vi "MoveZ.vi"(0 "Speed (unit/s)":dbl min=0.0 max=1500.0, 1 "Relative/Absolute\nPosition":enum16{"Relative", "Absolute"}(ring), 2 "connection refnum in":refnum<k5>, 5 "Speed Units":enum16{"mm", "µm"}(ring), 7 "Target Position":dbl, 9 "Target Units":enum16{"mm", "µm"}(ring), 11 "error in":errorcluster) -> (4 "connection refnum out z":refnum<k5>, 6 "approx move time (ms)":i32, 15 "error out":errorcluster)   [LabVIEW 2023]
doc: "Move in a fixed step to a target location in the Z direction"
uses:
  GlobalVarsNetwork.vi
panel:
  in  "Stop Button":bool
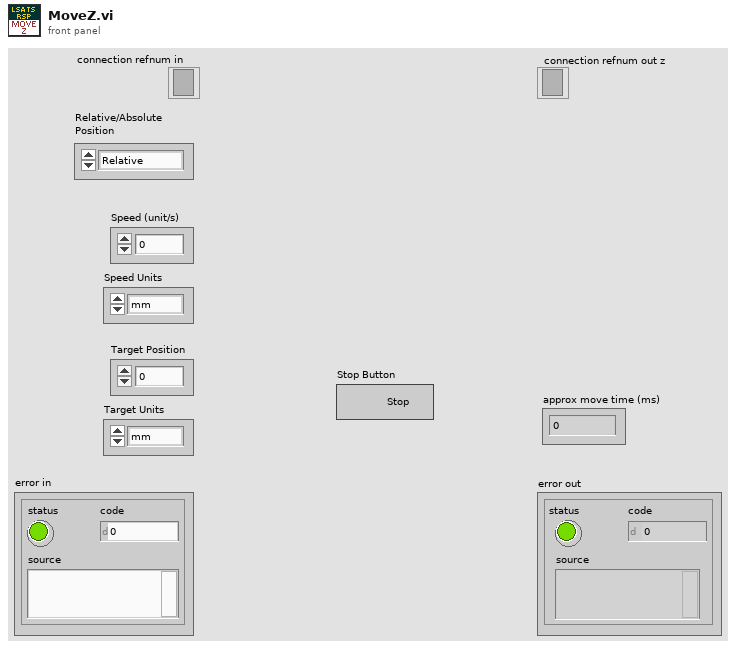
[diagram p1: front panel]
types:
  T1 = cluster{"XY_IP_ADDRESS":string, "Z_IP_ADDRESS":string, "Port":u16, "connection refnum x,y":refnum<k5>, "connection refnum z":refnum<k5>}
  T2 = enum8{"Enabled", "Disabled", "Disabled and Grayed Out"}
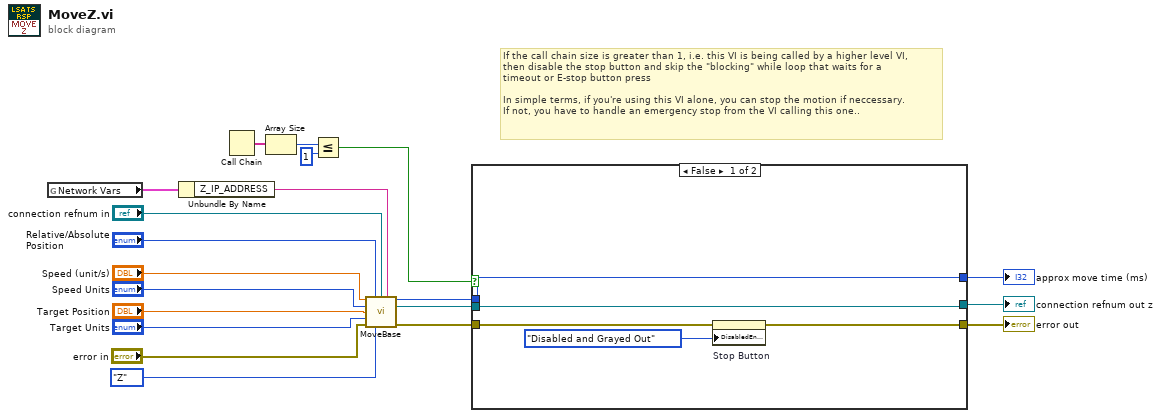
[diagram p0: block diagram]
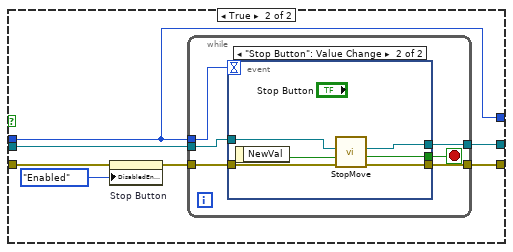
[diagram p2: hidden frame]
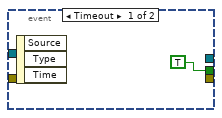
[diagram p3: hidden frame]
diagram:
  # "If the call chain size is greater than 1, i.e. this VI is being called by a higher level VI,\nthen disable the stop button and skip the \"blocking\" while loop that waits for a \ntimeout or E-stop button press\n\nIn simple terms, if you're using this VI alone, you can stop the motion if neccessary.\nIf not, you have to handle an emergency stop from the VI calling this one.."
  n1 = global read "GlobalVarsNetwork.vi" "Network Vars"() -> (w14:T1)
  n2 = Unbundle By Name(w14) -> ("Z_IP_ADDRESS"=w13:string)
  n3 = Call Chain() -> (call chain=w9:string[])
  n4 = Array Size(array=w9) -> (size(s)=w7:i32)
  n5 = Less Or Equal?(x=w7, y=1) -> (x <= y?=w6:bool)
  n6 = call "MoveBase.vi"("Speed"="Speed (unit/s)", "Relative/Absolute\nPosition"="Relative/Absolute\nPosition", "connection refnum in"="connection refnum in", "IP address"=w13, "Speed Units (unit/s)"="Speed Units", "Target Position"="Target Position", "Target Position Units"="Target Units", "error in"="error in", "Axis"=enum16{"Z", "Y", "X"}."Z") -> ("approx move time (ms)"=w10:i32, "connection refnum out"=w2:refnum<k5>, "error out"=w5:errorcluster)  [unwired: 4 in]
  n7 = case shown="False" w6 {
    tunnel: w5 -> [w25 w31]
    tunnel: [w24 w32] -> w11
    tunnel: w10 -> [w22 w28]
    tunnel: [w22 w28] -> w4
    tunnel: w2 -> [w21 w27]
    tunnel: [w21 w26] -> w1
    frame False {
      n8 = property on="Stop Button" class="Bool"(error in=w25, "DisabledEnum"=T2."Disabled and Grayed Out" ("Disabled")) -> (error out=w24:errorcluster)  [unwired: 1 in, 1 out]
    }
    frame True {
      n9 = property on="Stop Button" class="Bool"(error in=w31, "DisabledEnum"=T2."Enabled" ("Disabled")) -> (error out=w30:errorcluster)  [unwired: 1 in, 1 out]
      n10 = while {
        tunnel: w30 -> [w38]
        tunnel: [w37] -> w32
        tunnel: w28 -> [w35]
        tunnel: w27 -> [w34]
        tunnel: [w33] -> w26
        stop <- w36 stop-if-true
        n11 = event shown="[1] \"Stop Button\": Value Change" {
          selector: _ -> [_ _]
          dyn-events: _ -> [_ _]
          timeout: w35 -> [_ _]
          tunnel: w38 -> [_ w45]
          tunnel: [_ w44] -> w37
          tunnel: [TRUE w43] -> w36
          tunnel: w34 -> [_ w41]
          tunnel: [_ w40] -> w33
          event Timeout {
            n12 = event-data() -> ()  [unwired: 1 in, 3 out]
          }
          event "Stop Button": Value Change {
            n13 = event-data() -> ("NewVal"=w42:bool)  [unwired: 1 in]
            n14 = call "StopMove.vi"("error in"=w45, "Stop?"=w42, "connection refnum in,  z"=w41) -> ("error out"=w44:errorcluster, "Stop?"=w43:bool, "connection refnum out z"=w40:refnum<k5>)  [unwired: 1 in, 1 out]
          }
        }
      }
    }
  }
  "error out" <- w11
  "approx move time (ms)" <- w4
  "connection refnum out z" <- w1
